vi "Received Frame.vi"(8 "entrée d'erreur (pas d'erreur)":errorcluster, 11 "Send_Frame en entrée":refnum<class "Zigbee_Send_Command_UART.lvclass">) -> (0 "sortie d'erreur":errorcluster, 1 "Send again":bool, 2 "Frame read":string, 3 "Send_Frame en sortie":refnum<class "Zigbee_Send_Command_UART.lvclass">)   [LabVIEW 2020, in "Library Test.lvlib" / "Zigbee_Send_Command_UART.lvclass"]
uses:
  Zigbee_Send_Command_UART.lvclass
  C:/Users/ngarcin/OneDrive - Altyor/Standard TB/Class/Test/Test (Default)/Test (Default).lvclass
  JSON API/JSON Value/Set from JSON string.vi
  Instrument/Instrument (Default)/Class Instrument (Default).lvclass
  JSON API/JSON Value/JSON Value.lvclass
  Zigbee_Send_Command_UART.lvclass/Zigbee_Send_Command_UART.ctl
  JSON API/Variant JSON/Variant JSON.lvlib
  JSON API/Get Polymorphic/JSON GetSet.lvlib
  Commun VI/Library Commun.lvlib
  Test (Default)/Test (Default).lvclass
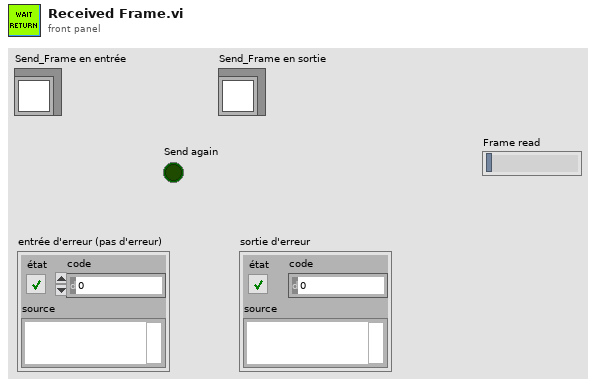
[diagram p1: front panel]
types:
  T1 = cluster{"Frame Read":string, "Frame received":bool, "Frame NOk":bool}
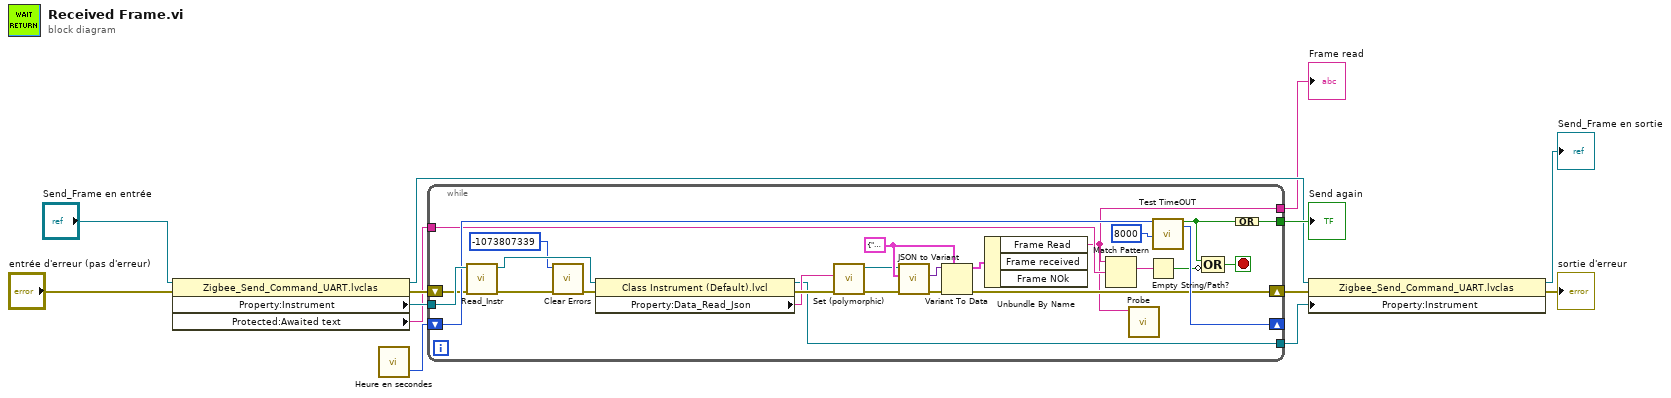
[diagram p0: block diagram]
diagram:
  n1 = property class="Zigbee_Send_Command_UART.lvclas"(reference="Send_Frame en entrée", error in="entrée d'erreur (pas d'erreur)") -> (reference out=w6:refnum<class "Zigbee_Send_Command_UART.lvclass">, error out=w3:errorcluster, "Property:Instrument"=w4:refnum<class "Class Instrument (Default).lvclass">, "Protected:Awaited text"=w1:string)
  n2 = call "Heure en secondes.vi"() -> ("Heure en milisecondes"=w5:u32)  [unwired: 2 in, 1 out]
  n3 = while {
    tunnel: w4 -> [w30]
    shift-right: [w24] -> w10
    shift-left: w3 -> [w21]
    tunnel: [w29] -> w7
    shift-right: [w27] -> _
    shift-left: w5 -> [w28]
    tunnel: [w25] -> w13
    tunnel: [w14] -> w2
    tunnel: w1 -> [w15]
    stop <- w22 stop-if-true
    w38 = T1 {"Frame Read"="", "Frame received"=FALSE, "Frame NOk"=FALSE}
    n4 = call-dynamic "Read_Instr.vi"("error in (no error)"=w21, "Class Instrument (Default) en entrée"=w30) -> ("error out"=w20:errorcluster, "Class Instrument (Default) en sortie"=w31:refnum<class "Class Instrument (Default).lvclass">)  [unwired: 8 in]
    n5 = call <vilib>:"Clear Errors.vi"("error in (no error)"=w20, "specific error code to clear (0: all)"=-1073807339) -> ("error out"=w18:errorcluster)  [unwired: 4 in, 1 out]
    n6 = property class="Class Instrument (Default).lvcl"(reference=w31, error in=w18) -> (reference out=w29:refnum<class "Class Instrument (Default).lvclass">, error out=w36:errorcluster, "Property:Data_Read_Json"=w35:string)
    n7 = call-poly "Set (polymorphic).vi"("error in (no error)"=w36, "JSON stream"=w35) -> ("error out"=w32:errorcluster, "JSON Value out"=w34:refnum<class "JSON Value.lvclass">)  [unwired: 7 in, 1 out]
    n8 = call "JSON to Variant.vi"("error in (no error)"=w32, "Variant (Data Type)"=w38, "JSON Value"=w34) -> ("error out"=w33:errorcluster, "Variant out"=w37:variant)  [unwired: 7 in]
    n9 = Variant To Data(error in=w33, type=w38, Variant=w37) -> (data=w39:T1, error out=w24:errorcluster)
    n10 = Unbundle By Name(w39) -> ("Frame Read"=w14:string)  [unwired: 2 out]
    n11 = Match Pattern(string=w14, regular expression=w15) -> (match substring=w17:string)  [unwired: 1 in, 3 out]
    n12 = call "Probe.vi"("Message"=w14) -> ()  [unwired: 10 in, 1 out]
    n13 = Empty String/Path?(string/path=w17) -> (empty?=w16:bool)
    n14 = call "Test TimeOUT.vi"("OLD Time"=w28, "TimeOut ms"=u32 8000) -> ("Timeout ?"=w23:bool, "NEW Time"=w27:u32)  [unwired: 13 in, 3 out]
    n15 = Compound Arithmetic op=OR ("Opérateur arithmétique")(w23, invert w16) -> (w22:bool)
    n16 = Compound Arithmetic op=OR ("Opérateur arithmétique")(w23) -> (w25:bool)
  }
  "Frame read" <- w2
  "Send again" <- w13
  n17 = property class="Zigbee_Send_Command_UART.lvclas"(reference=w6, error in=w10, "Property:Instrument"=w7) -> (reference out=→"Send_Frame en sortie":refnum<class "Zigbee_Send_Command_UART.lvclass">, error out=→"sortie d'erreur":errorcluster)
